vi "setAttribute_Number_Int16.vi"(7 "object":string, 8 "error in (no error)":errorcluster, 9 "data":i16, 10 "attribute":string, 11 "LabVIEW-Python-Interface in":refnum<class "PyLVi.lvclass">) -> (0 "error out":errorcluster, 3 "LabVIEW-Python-Interface out":refnum<class "PyLVi.lvclass">)   [LabVIEW 2016, in "PyLVi.lvlib" / "PyLVi.lvclass"]
uses:
  PyLVi.lvclass
  argument_add/addArgument_Number_Int16.vi
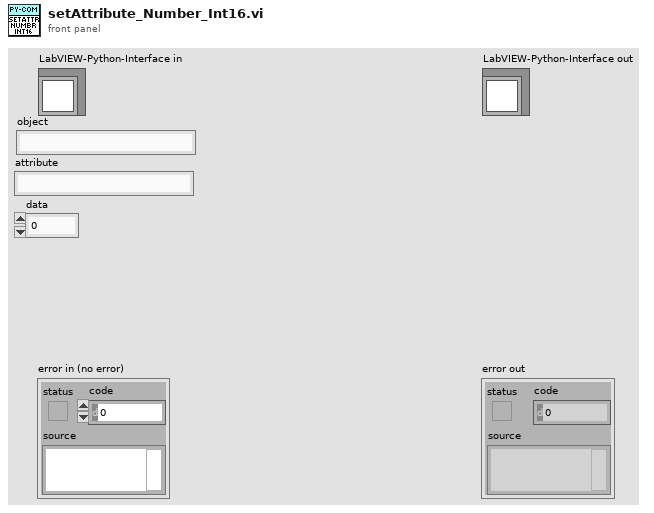
[diagram p1: front panel]
types:
  T1 = typedef "PyLVi.lvlib/PyLVi.lvclass/ArgumentStructure.ctl" = cluster{"descriptor structure":T2, "data string":string}
  T2 = typedef "PyLVi.lvlib/PyLVi.lvclass/DescriptorStructure.ctl" = cluster{"argtype":string, "dtype":string, "shape":u32[], "argname":string}
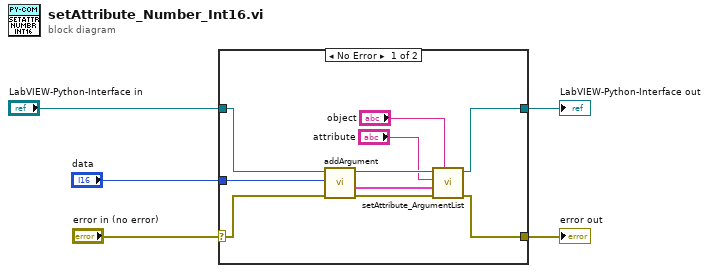
[diagram p0: block diagram]
diagram:
  n1 = case shown="No Error" "error in (no error)" {
    selector: "error in (no error)" -> [w9 w17]
    tunnel: [w8 w17] -> w4
    tunnel: [w7 w16] -> w2
    tunnel: "LabVIEW-Python-Interface in" -> [w15 w16]
    tunnel: "data" -> [w6 _]
    frame No Error {
      n2 = call-poly "addArgument.vi"("error in (no error)"=w9, "data"=w6, "LabVIEW-Python-Interface in"=w15) -> ("error out"=w10:errorcluster, "argument list out"=w13:T1[], "LabVIEW-Python-Interface out"=w14:refnum<class "PyLVi.lvclass">)  [unwired: 6 in]
      n3 = call "setAttribute_ArgumentList.vi"("object"="object", "error in (no error)"=w10, "argument list in"=w13, "attribute"="attribute", "LabVIEW-Python-Interface in"=w14) -> ("error out"=w8:errorcluster, "LabVIEW-Python-Interface out"=w7:refnum<class "PyLVi.lvclass">)  [unwired: 4 in, 1 out]
    }
    frame Error {
    }
  }
  "error out" <- w4
  "LabVIEW-Python-Interface out" <- w2
